vi "Units_DegreesToRadians.vi"(10 "Degrees":dbl) -> (2 "Radians":dbl)   [LabVIEW 2019, in "Trajectory_Library.lvlib"]
doc: "Convert Meters to Feet"
uses:
  Trajectory_Library.lvlib
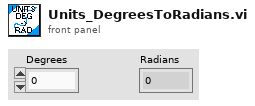
[diagram p1: front panel]
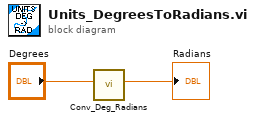
[diagram p0: block diagram]
diagram:
  n1 = call "Conv_Deg_Radians.vi"("Degress"="Degrees") -> ("Radians"=→"Radians":dbl)  [unwired: 10 in]
